vi "Publish Counter.vi"(8 "error in":errorcluster, 10 "Counter Data":dbl[](array[numeric]), 11 "BNT_ULx-MCSV in":refnum<class "BNT_ULx-MCSV.lvclass">) -> (0 "error out":errorcluster, 3 "BNT_ULx-MCSV out":refnum<class "BNT_ULx-MCSV.lvclass">)   [LabVIEW 2021, in "BNT_ULx.lvlib" / "BNT_ULx-MCSV.lvclass"]
doc: "Publish counter values if changed."
uses:
  BNT_ULx-MCSV.lvclass
  BNT_ULx-MCSV.lvclass/BNT_ULx-MCSV.ctl
  CSPP_Core/Classes/CSPP_ProcessVariables/PVConnection/PVConnection.lvclass/PVConnection.ctl
  CSPP_Core/Classes/CSPP_ProcessVariables/ProcessVariable/PV.lvclass/PV.ctl
  CSPP_Core/Classes/CSPP_ProcessVariables/ProcessVariable/Write Data.vi
  CSPP_Core/Classes/CSPP_ProcessVariables/ProcessVariable/Write Error.vi
  CSPP_Core/Classes/CSPP_ProcessVariables/ProcessVariable/Write Quality.vi
  CSPP_Core/Classes/CSPP_ProcessVariables/ProcessVariable/Write status.vi
  CSPP_Core/Classes/CSPP_ProcessVariables/ProcessVariable/Write Timestamp.vi
  CSPP_Core/Classes/CSPP_ProcessVariables/ProcessVariable/PV.lvclass
  CSPP_Core/Classes/CSPP_ProcessVariables/PVConnection/PVConnection.lvclass
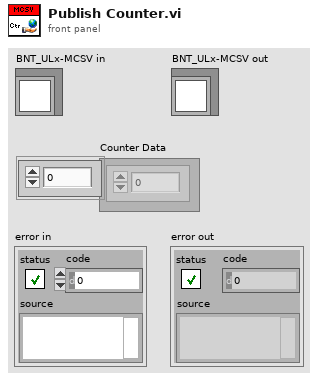
[diagram p1: front panel]
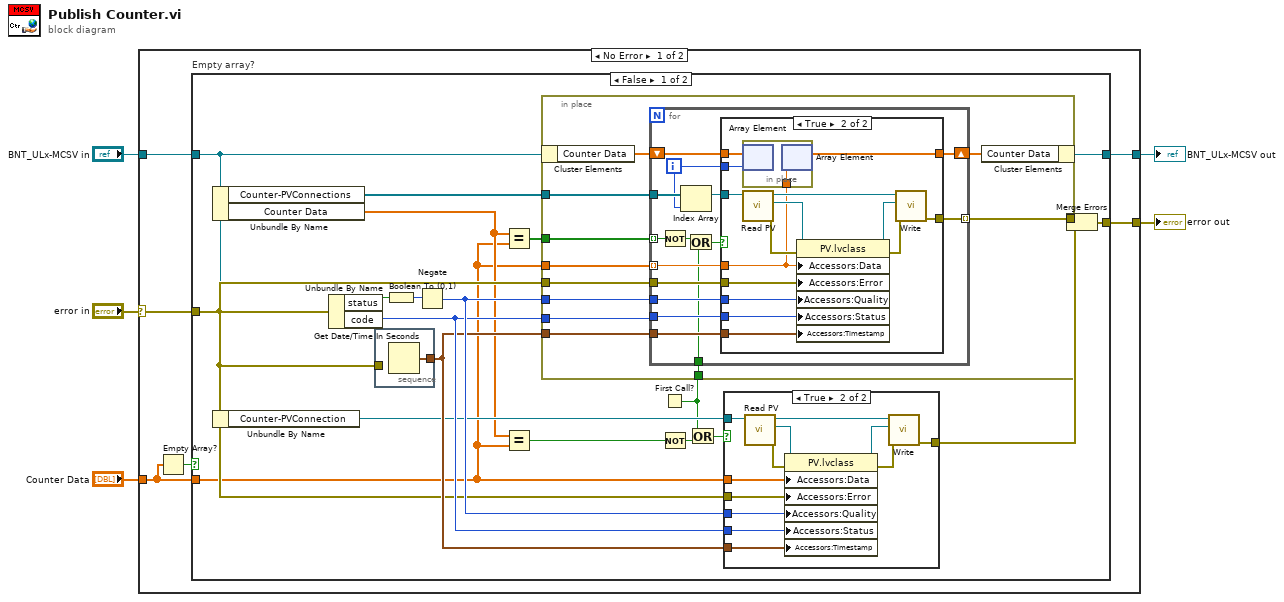
[diagram p0: block diagram]
diagram:
  n1 = case shown="No Error" "error in" {
    selector: "error in" -> [w11 w93]
    tunnel: [w10 w93] -> w4
    tunnel: [w8 w92] -> w2
    tunnel: "BNT_ULx-MCSV in" -> [w9 w92]
    tunnel: "Counter Data" -> [w6 _]
    frame No Error {
      n2 = Empty Array?(array=w6) -> (empty?=w7:bool)
      n3 = case "Empty array?" shown="False" w7 {
        tunnel: w11 -> [w24 w90]
        tunnel: [w22 w90] -> w10
        tunnel: w6 -> [w14 _]
        tunnel: w9 -> [w18 w91]
        tunnel: [w17 w91] -> w8
        frame False {
          n4 = Unbundle By Name(w18) -> ("Counter-PVConnections"=w23:refnum<class "PVConnection.lvclass">[], "Counter Data"=w19:dbl[])
          n5 = Unbundle By Name(w18) -> ("Counter-PVConnection"=w21:refnum<class "PVConnection.lvclass">)
          n6 = Unbundle By Name(w24) -> ("status"=w30:bool, "code"=w27:i32)
          n7 = stacked-sequence {
            tunnel: [w32] -> w26
            tunnel: w24 -> [_]
            frame #0 {
              n8 = Get Date/Time In Seconds() -> (seconds since 1Jan1904=w32:timestamp)
            }
          }
          n9 = Boolean To (0,1)(Boolean=w30) -> (0, 1=w29:i16)
          n10 = Negate(x=w29) -> (-x=w28:i16)
          n11 = Equal?(x=w19, y=w14) -> (x = y?=w20:bool[])
          n12 = Equal?(x=w19, y=w14) -> (x = y?=w16:bool)
          n13 = First Call?() -> (First Call?: T/F=w13:bool)
          n14 = in-place {
            in-place-border: [w43] -> w31
            in-place-border: w28 -> [w42]
            in-place-border: w27 -> [w41]
            in-place-border: w26 -> [w40]
            in-place-border: w24 -> [w39]
            in-place-border: w23 -> [w38]
            in-place-border: w14 -> [w37]
            in-place-border: w20 -> [w36]
            in-place-border: w13 -> [w33]
            n15 = in-place-cluster #1(w18) -> ("Counter Data"=w35:dbl[])
            n16 = for {
              tunnel: w38 -> [w52]
              tunnel: w37 -> [w58] mode=indexing
              tunnel: w39 -> [w57]
              tunnel: [w56] -> w43 mode=indexing
              tunnel: w42 -> [w55]
              tunnel: w41 -> [w54]
              tunnel: w40 -> [w53]
              tunnel: w36 -> [w51] mode=indexing
              shift-right: [w49] -> w34
              shift-left: w35 -> [w50]
              tunnel: w33 -> [w47]
              i -> [w44]
              n17 = Not(x=w51) -> (.not. x?=w46:bool)
              n18 = Index Array(array=w52, index=w44) -> (element=w45:refnum<class "PVConnection.lvclass">)
              n19 = Or(x=w46, y=w47) -> (x .or. y?=w48:bool)
              n20 = case shown="True" w48 {
                tunnel: w58 -> [_ w62]
                tunnel: w57 -> [w60 w75]
                tunnel: [w60 w72] -> w56
                tunnel: w55 -> [_ w71]
                tunnel: w54 -> [_ w70]
                tunnel: w53 -> [_ w69]
                tunnel: w45 -> [_ w68]
                tunnel: w44 -> [_ w64]
                tunnel: w50 -> [w59 w63]
                tunnel: [w59 w61] -> w49
                frame False {
                }
                frame True {
                  n21 = in-place {
                    in-place-border: w62 -> [w76]
                    n22 = in-place-array #2(w63, w64) -> ()  [unwired: 1 out]
                    n23 = in-place-array #2(w76) -> (w61:dbl[])  [unwired: 1 out]
                  }
                  n24 = call "Read PV.vi"("PVConnection in"=w68) -> ("error out"=w65:errorcluster, "PV"=w66:refnum<class "PV.lvclass">, "PVConnection out"=w67:refnum<class "PVConnection.lvclass">)  [unwired: 8 in]
                  n25 = property class="PV.lvclass"(reference=w66, error in=w65, "Accessors:Data"=w62, "Accessors:Error"=w75, "Accessors:Quality"=w71, "Accessors:Status"=w70, "Accessors:Timestamp"=w69) -> (reference out=w74:refnum<class "PV.lvclass">, error out=w73:errorcluster)
                  n26 = call "Write.vi"("error in (no error)"=w73, "PV"=w74, "PVConnection in"=w67) -> ("error out"=w72:errorcluster)  [unwired: 6 in, 2 out]
                }
              }
            }
            n27 = in-place-cluster #1("Counter Data"=w34) -> (w17:refnum<class "BNT_ULx-MCSV.lvclass">)
          }
          n28 = Not(x=w16) -> (.not. x?=w12:bool)
          n29 = Or(x=w13, y=w12) -> (x .or. y?=w15:bool)
          n30 = case shown="True" w15 {
            tunnel: w28 -> [_ w84]
            tunnel: w27 -> [_ w83]
            tunnel: w26 -> [_ w82]
            tunnel: [w77 w81] -> w25
            tunnel: w24 -> [w77 w80]
            tunnel: w21 -> [_ w79]
            tunnel: w14 -> [_ w78]
            frame False {
            }
            frame True {
              n31 = call "Read PV.vi"("PVConnection in"=w79) -> ("error out"=w85:errorcluster, "PV"=w86:refnum<class "PV.lvclass">, "PVConnection out"=w87:refnum<class "PVConnection.lvclass">)  [unwired: 8 in]
              n32 = property class="PV.lvclass"(reference=w86, error in=w85, "Accessors:Data"=w78, "Accessors:Error"=w80, "Accessors:Quality"=w84, "Accessors:Status"=w83, "Accessors:Timestamp"=w82) -> (reference out=w89:refnum<class "PV.lvclass">, error out=w88:errorcluster)
              n33 = call "Write.vi"("error in (no error)"=w88, "PV"=w89, "PVConnection in"=w87) -> ("error out"=w81:errorcluster)  [unwired: 6 in, 2 out]
            }
          }
          n34 = Merge Errors(w31, w25) -> (w22:errorcluster)
        }
        frame True {
        }
      }
    }
    frame Error {
    }
  }
  "error out" <- w4
  "BNT_ULx-MCSV out" <- w2
